vi "BasicOfNotifier.vi"() -> ()   [LabVIEW 2020]
doc: "This VI demonstrates basic concepst of notifiers in LabVIEW. Comments in Polish."
panel:
  out "Notifier name":string
  out "Last notification":i32
  out "Error Out":errorcluster
  out "CanceldNoti":i32
  out "Noti4":i32
  out "T_Out2":bool caption="Timed out!"
  out "T_Out1":bool caption="Timed out!"
  out "Noti3":i32
  out "Noti2":i32=3
  out "Noti1":i32
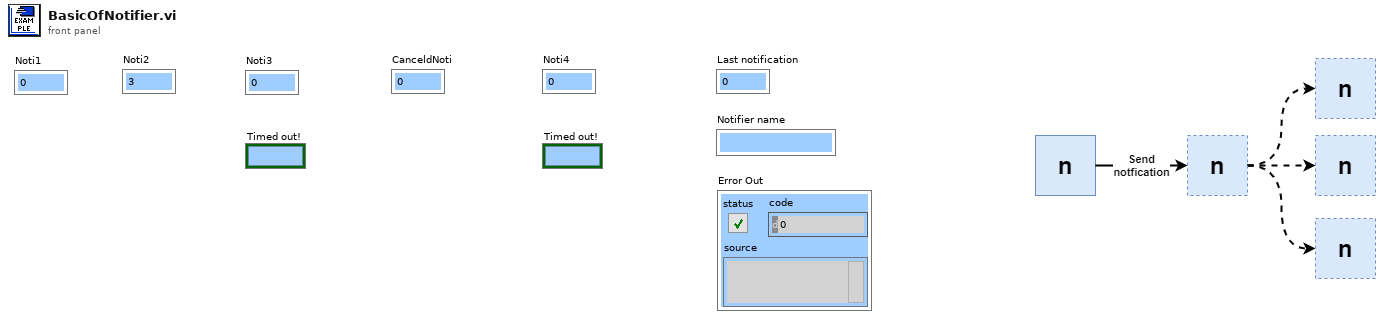
[diagram p1: front panel]
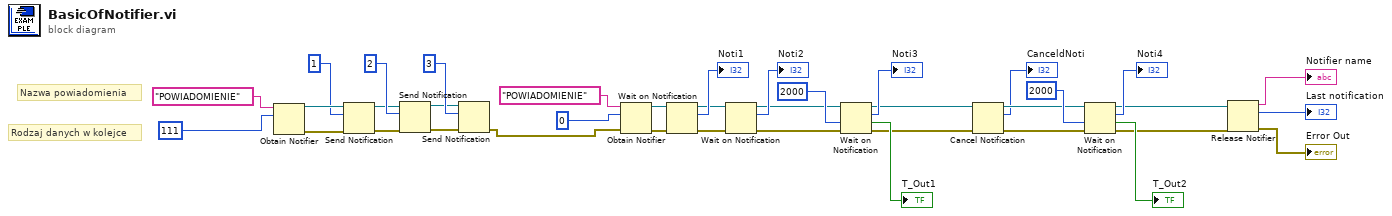
[diagram p0: block diagram]
diagram:
  # "Rodzaj danych w kolejce"
  # "Nazwa powiadomienia"
  n1 = Obtain Notifier(name (unnamed)="POWIADOMIENIE", notification data type=111) -> (notifier out=w36:refnum<notifier>, error out=w35:errorcluster)  [unwired: 2 in, 1 out]
  n2 = Send Notification(notification=1, notifier=w36, error in (no error)=w35) -> (notifier out=w31:refnum<notifier>, error out=w32:errorcluster)
  n3 = Send Notification(notification=2, notifier=w31, error in (no error)=w32) -> (notifier out=w29:refnum<notifier>, error out=w28:errorcluster)
  n4 = Send Notification(notification=3, notifier=w29, error in (no error)=w28) -> (error out=w25:errorcluster)  [unwired: 1 out]
  n5 = Obtain Notifier(name (unnamed)="POWIADOMIENIE", notification data type=0, error in (no error)=w25) -> (notifier out=w23:refnum<notifier>, error out=w24:errorcluster)  [unwired: 1 in, 1 out]
  n6 = Wait on Notification(notifier=w23, error in (no error)=w24) -> (notifier out=w20:refnum<notifier>, notification=→"Noti1":i32, error out=w19:errorcluster)  [unwired: 2 in, 1 out]
  n7 = Wait on Notification(notifier=w20, error in (no error)=w19) -> (notifier out=w16:refnum<notifier>, notification=→"Noti2":i32, error out=w15:errorcluster)  [unwired: 2 in, 1 out]
  n8 = Wait on Notification(notifier=w16, timeout in ms (-1)=2000, error in (no error)=w15) -> (notifier out=w8:refnum<notifier>, notification=→"Noti3":i32, timed out?=→"T_Out1":bool, error out=w10:errorcluster)  [unwired: 1 in]
  n9 = Cancel Notification(0:w8, 3:w10) -> (8:w7:refnum<notifier>, 9:→"CanceldNoti":i32, 11:w9:errorcluster)
  n10 = Wait on Notification(notifier=w7, timeout in ms (-1)=2000, error in (no error)=w9) -> (notifier out=w4:refnum<notifier>, notification=→"Noti4":i32, timed out?=→"T_Out2":bool, error out=w5:errorcluster)  [unwired: 1 in]
  n11 = Release Notifier(notifier=w4, error in (no error)=w5) -> (notifier name=→"Notifier name":string, last notification=→"Last notification":i32, error out=→"Error Out":errorcluster)  [unwired: 1 in]
